vi "一体站流程自动启动.vi"(11 "参数":T1) -> ()   [LabVIEW 2016, in "PLC.lvlib"]
uses:
  PLC.lvlib
panel:
  out "s? t:f":enum16{"初始化", "采配水启动", "仪器操作", "反冲洗", "结束"}(ring)
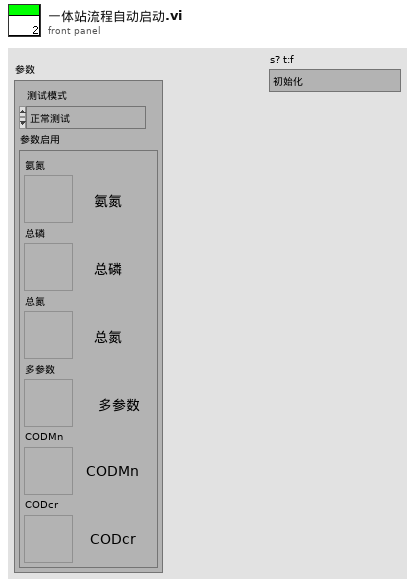
[diagram p1: front panel]
types:
  T1 = cluster{"测试模式":enum16{"正常测试", "集成干预"}, "参数启用":cluster{"氨氮":bool, "总磷":bool, "总氮":bool, "多参数":bool, "CODMn":bool, "CODcr":bool}}
  T2 = cluster{"命令":string, cluster{"starting address":u16, "holding register value":u16}}
  T3 = enum16{"启动测量", "标样核查", "零点核查", "跨度核查", "空白测试", "平行样测试", "加标回收", "空白校准", "标样校准", "初始化（清洗）", "停止测试", "仪器重启", "校时", "模式设置", "测量间隔设置"}
  T4 = cluster{"时间标识":timestamp, "设备":string, "日志信息":string, "流程参数":string}
  T5 = cluster{"测量模式":enum16{"水样测量", "标样核查", "零点核查", "跨度核查", "空白测试", "加标回收", "平行样", "校零", "校标"}}
  T6 = cluster{"时间标识":timestamp, "设备":string, "日志信息":string}
  T7 = enum16{"空闲", "水样测试", "标样核查", "零点核查", "跨度核查", "空白测试", "平行样测试", "加标回收", "空白校准", "标样校准", "初始化（清洗）"}
  T8 = cluster{"R0":i16, "R1":i16, "R2":i16, "R3":i16, "R4":i16, "R5":i16, "R6":i16, "R7":i16, "R8":i16, "R9":i16, "R10":i16, "R11":i16, "R12":i16, "R13":i16, "R14":i16, "R15":i16, "R16":i16, "R17":i16, "R18":i16, "R19":i16, "R20":i16, "R21":i16, "R22":i16, "R23":i16, "R24":i16, "R25":i16, "R26":i16, "R27":i16, "R28":i16, "R29":i16, "R30":i16, "R31":i16}
  T9 = cluster{"R100":i16, "R101":i16, "R102":i16, "R103":i16, "R104":i16, "R105":i16, "R106":i16, "R107":i16, "R108":i16, "R109":i16, "R110":i16, "R111":i16, "R112":i16, "R113":i16, "R114":i16, "R115":i16, "R116":i16, "R117":i16, "R118":i16, "R119":i16}
  T10 = enum32{"Bad", "Idle", "Run top level", "Running"}
  T11 = cluster{"氨氮":bool, "总磷":bool, "总氮":bool, "多参数":bool, "CODMn":bool, "CODcr":bool}
  T12 = cluster{"时间标识":timestamp, "参数":string, "集成干预测试浓度值":dbl, "集成干预前测试时间":timestamp, "集成干预前测试浓度值":dbl}
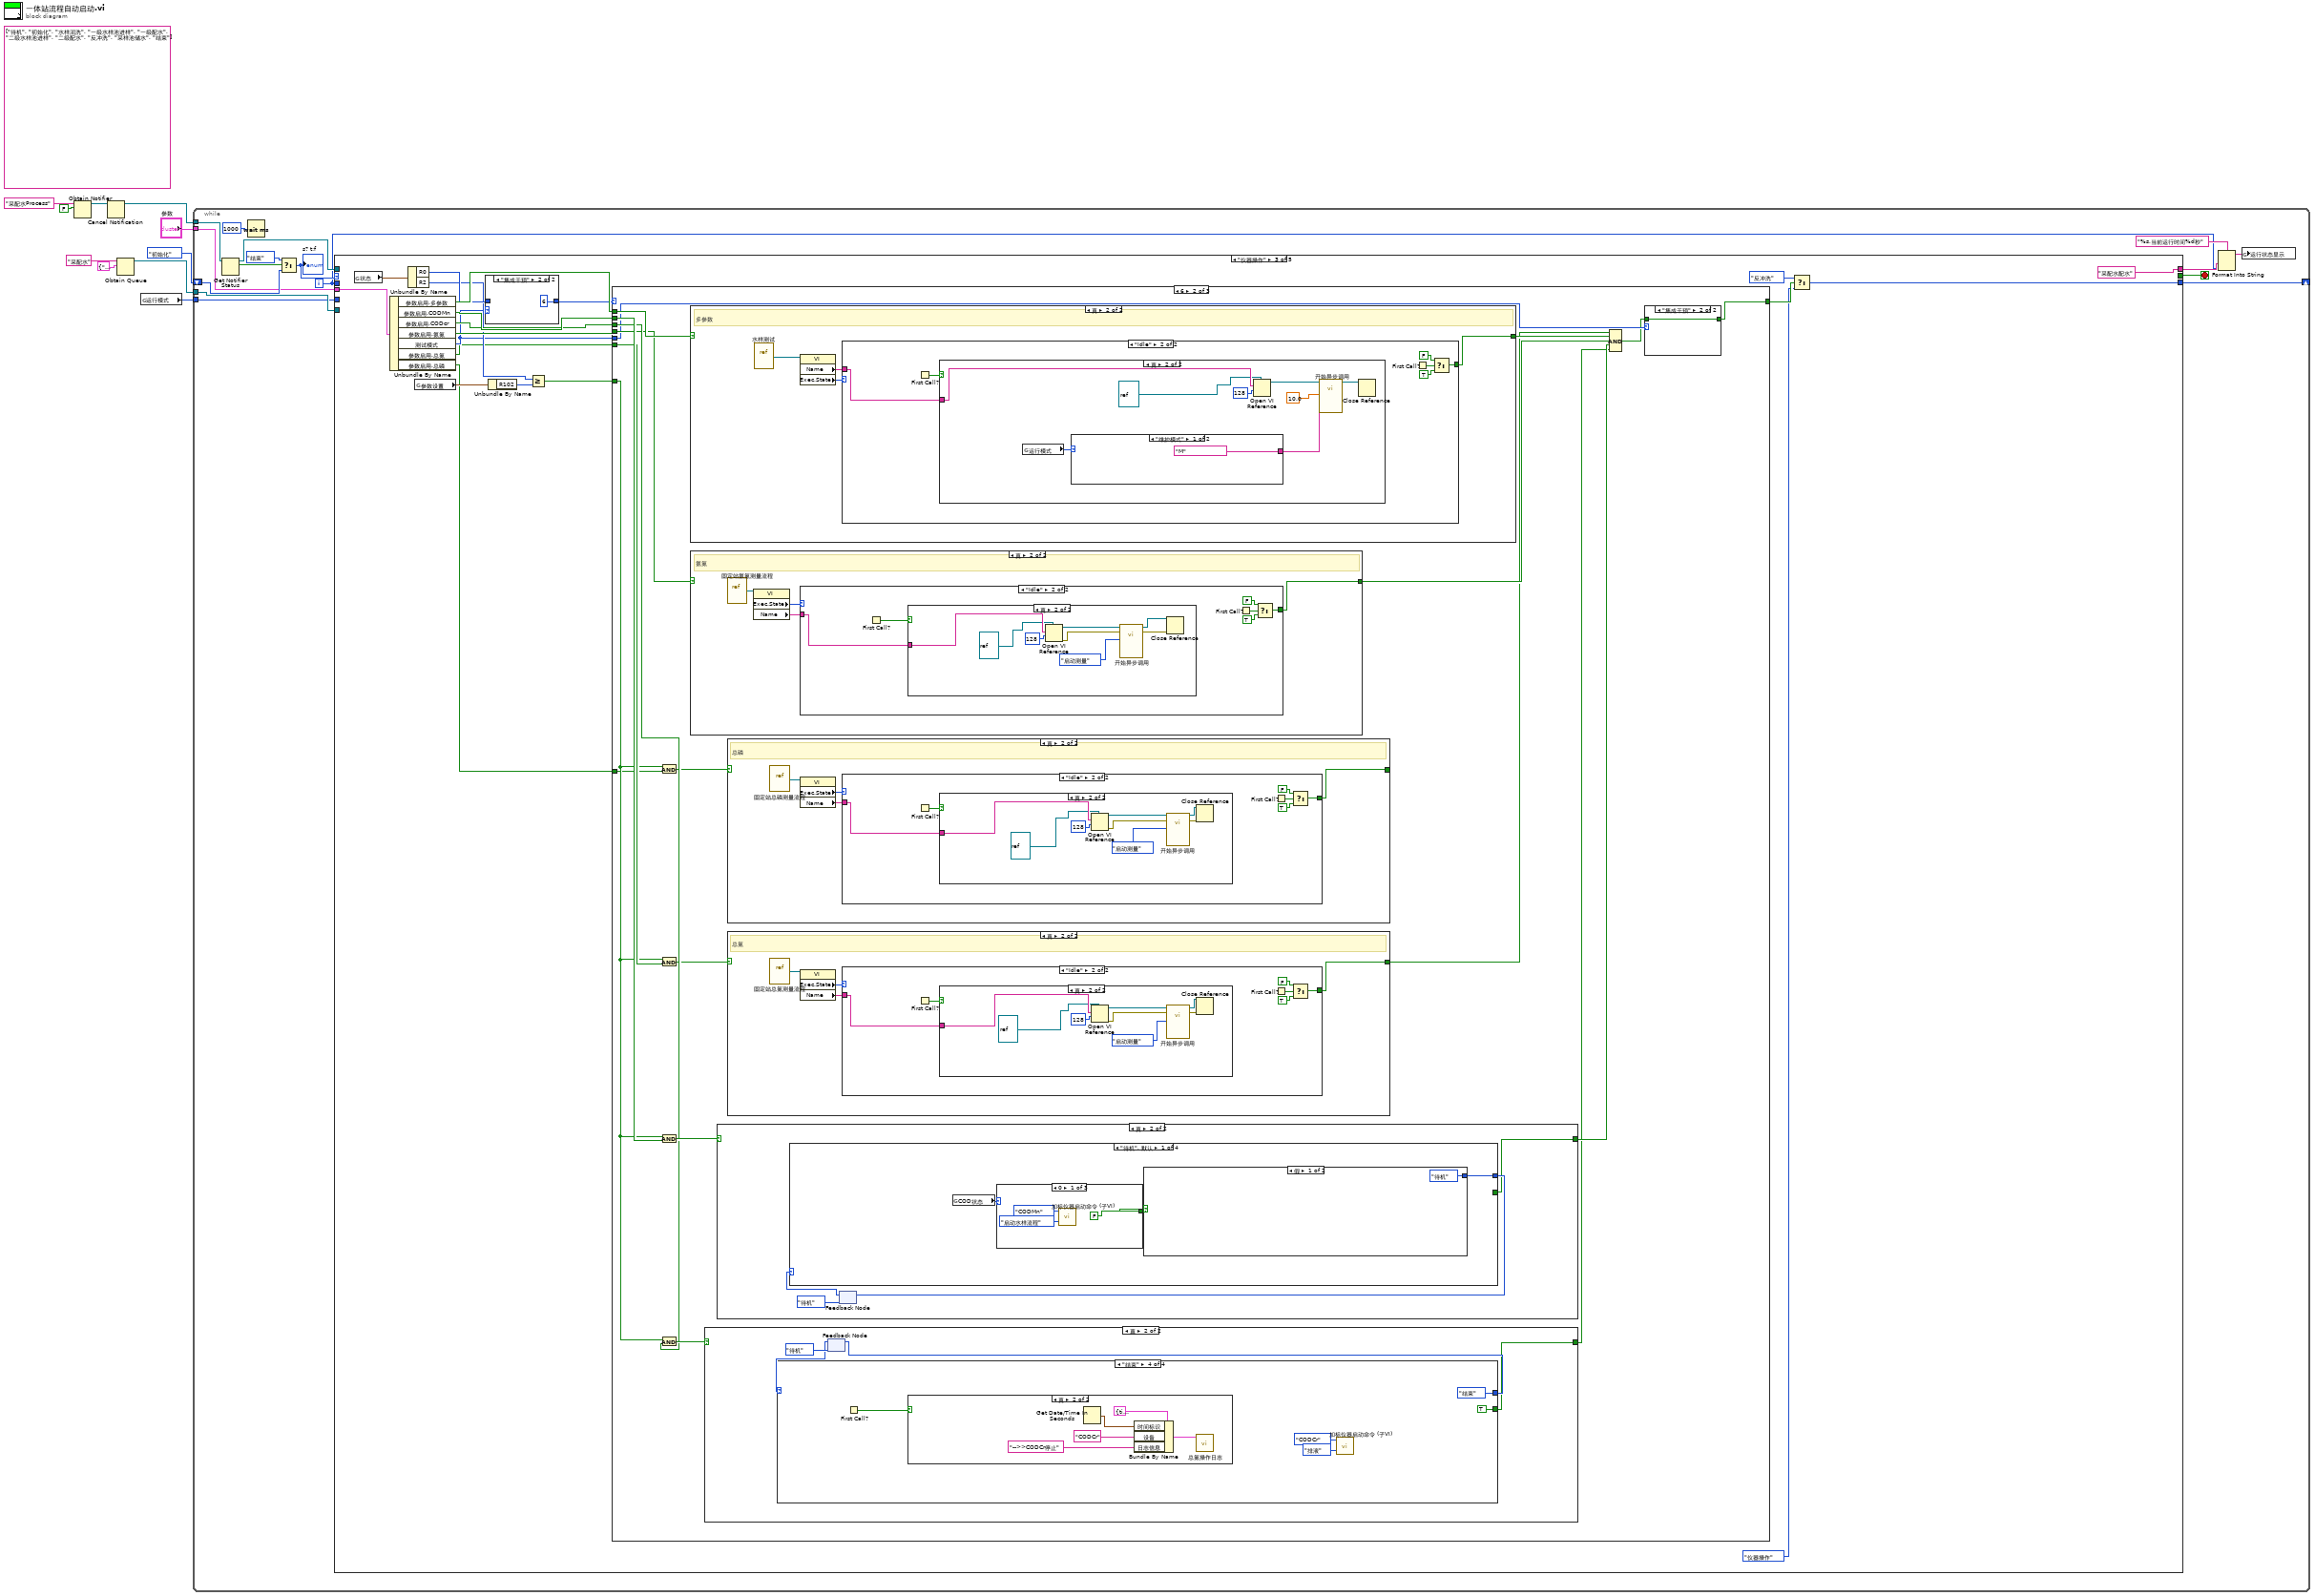
[diagram p0: block diagram]
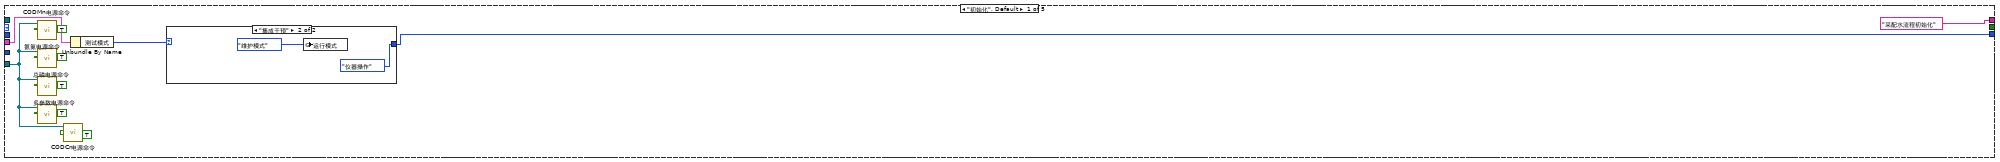
[diagram p2: hidden frame]
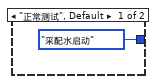
[diagram p3: hidden frame]
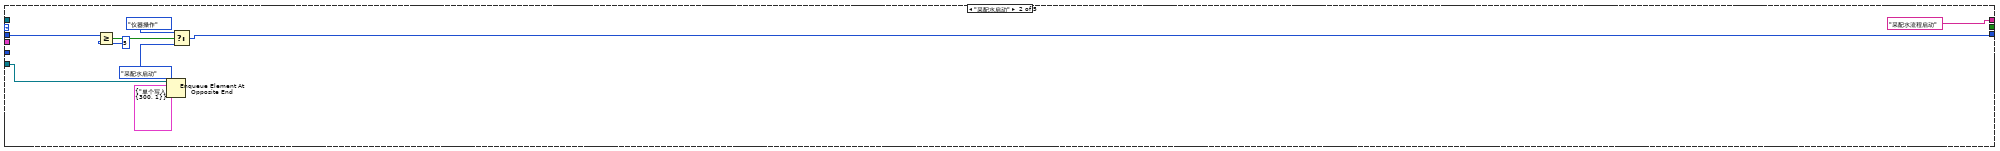
[diagram p4: hidden frame]
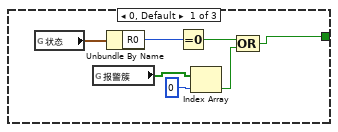
[diagram p6: hidden frame]
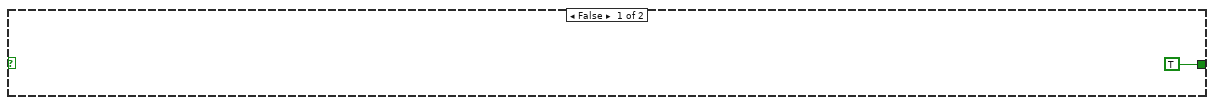
[diagram p7: hidden frame]
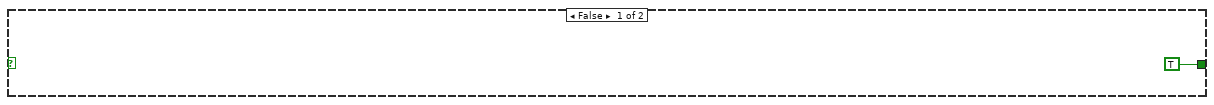
[diagram p10: hidden frame]
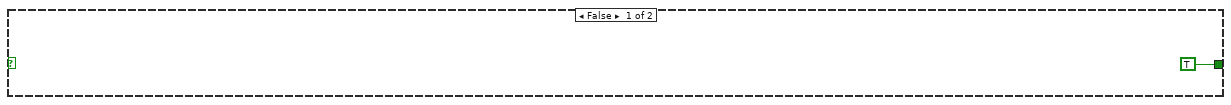
[diagram p14: hidden frame]
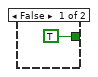
[diagram p17: hidden frame]
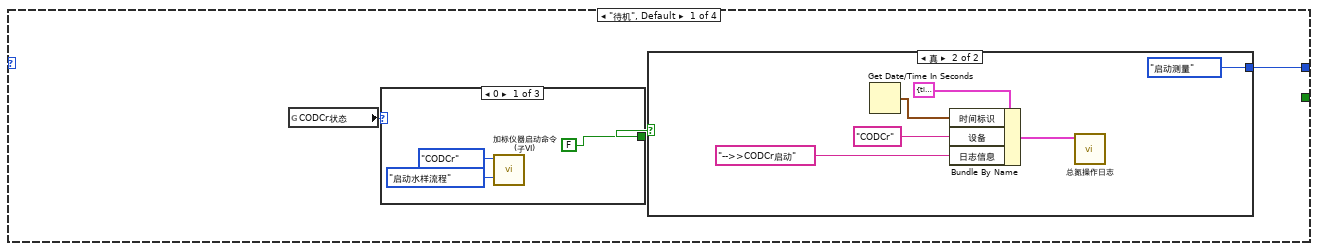
[diagram p18: hidden frame]
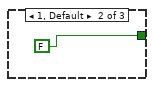
[diagram p19: hidden frame]
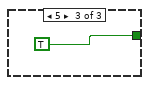
[diagram p20: hidden frame]
diagram:
  (unwired) string[][] [["待机"], ["初始化"], ["水样润洗"], ["一级水样池进样"], ["一级配水"], ["二级水样池进样"], ["二级配水"], ["反冲洗"], ["采样池储水"], ["结束"]] ("项名")
  n1 = Obtain Notifier(name (unnamed)="采配水Process" ("名称（未命名）"), notification data type=FALSE) -> (notifier out=w4:refnum<notifier>)  [unwired: 2 in, 2 out]
  n2 = Cancel Notification(0:w4) -> (8:w3:refnum<notifier>)  [unwired: 1 in, 2 out]
  n3 = Obtain Queue(name (unnamed)="采配水" ("名称（未命名）"), element data type=cluster{"命令":string, "数据":variant} {"命令"="", "数据"=variant}) -> (queue out=w7:refnum<queue>)  [unwired: 3 in, 2 out]
  n4 = global read "系统设置全局变量.vi" "运行模式"() -> (w1:enum16{"维护模式", "常规模式", "应急模式", "质控模式"})
  n5 = while {
    shift-right: [w23] -> _
    shift-left: enum16{"初始化", "采配水启动", "仪器操作", "反冲洗", "结束"}."初始化" ("枚举") -> [w19]
    tunnel: w7 -> [w26]
    tunnel: w3 -> [w22]
    tunnel: "参数" -> [w13]
    tunnel: w1 -> [w12]
    i -> [w11]
    stop <- w25 stop-if-true
    n6 = Get Notifier Status(notifier=w22) -> (notifier out=w14:refnum<notifier>, current notification=w21:bool)  [unwired: 1 in, 3 out]
    n7 = Wait (ms)(milliseconds to wait=u32 1000 ("等待时间（毫秒）")) -> ()  [unwired: 1 out]
    n8 = Select(t=enum16{"初始化", "采配水启动", "仪器操作", "反冲洗", "结束"}."结束" ("枚举"), s=w21, f=w19) -> (s? t:f=w18:enum16{"初始化", "采配水启动", "仪器操作", "反冲洗", "结束"})
    "s? t:f" <- w18
    n9 = case shown="\"仪器操作\"" w18 {
      tunnel: w26 -> [w31 w48 _ _ w473]
      tunnel: [_ _ _ _ TRUE] -> w25
      tunnel: [w30 w40 w63 w305 enum16{"初始化", "采配水启动", "仪器操作", "反冲洗", "结束"}."结束" ("枚举")] -> w23
      tunnel: ["采配水流程初始化" "采配水流程启动" "采配水配水" "等待测试完成" "采配水结束"] -> w15
      tunnel: w14 -> [_ _ _ _ w474]
      tunnel: w13 -> [w28 _ w66 w304 w470]
      tunnel: w12 -> [_ _ _ _ w469]
      tunnel: w11 -> [_ w46 _ _ _]
      frame "初始化", Default {
        n10 = call "CODMn电源命令.vi"("通电/断电"=TRUE, "队列"=w31) -> ()  [unwired: 9 in, 1 out]
        n11 = call "氨氮电源命令.vi"("通电/断电"=TRUE, "队列"=w31) -> ()  [unwired: 9 in, 1 out]
        n12 = call "总磷电源命令.vi"("通电/断电"=TRUE, "队列"=w31) -> ()  [unwired: 9 in, 1 out]
        n13 = call "多参数电源命令.vi"("通电/断电"=TRUE, "队列"=w31) -> ()  [unwired: 9 in, 1 out]
        n14 = call "CODCr电源命令.vi"("通电/断电"=TRUE, "队列"=w31) -> ()  [unwired: 9 in, 1 out]
        n15 = Unbundle By Name(w28) -> ("测试模式"=w27:enum16{"正常测试", "集成干预"})
        n16 = case shown="\"集成干预\"" w27 {
          tunnel: [enum16{"初始化", "采配水启动", "仪器操作", "反冲洗", "结束"}."采配水启动" ("枚举") enum16{"初始化", "采配水启动", "仪器操作", "反冲洗", "结束"}."仪器操作" ("枚举")] -> w30
          frame "正常测试", Default {
          }
          frame "集成干预" {
            n17 = global write "系统设置全局变量.vi" "运行模式"(enum16{"维护模式", "常规模式", "应急模式", "质控模式"}."维护模式" ("运行模式")) -> ()
          }
        }
      }
      frame "采配水启动" {
        n18 = Greater Or Equal?(x=w46, y=5) -> (x >= y?=w43:bool)
        n19 = Enqueue Element At Opposite End(queue=w48, element=T2 {"命令"="单个写入", {"starting address"=300, "holding register value"=1}} ("元素")) -> ()  [unwired: 2 in, 3 out]
        n20 = Select(t=enum16{"初始化", "采配水启动", "仪器操作", "反冲洗", "结束"}."仪器操作" ("枚举"), s=w43, f=enum16{"初始化", "采配水启动", "仪器操作", "反冲洗", "结束"}."采配水启动" ("枚举")) -> (s? t:f=w40:enum16{"初始化", "采配水启动", "仪器操作", "反冲洗", "结束"})
      }
      frame "仪器操作" {
        n21 = global read "采配水全局变量.vi" "状态"() -> (w68:T8)
        n22 = Unbundle By Name(w66) -> ("参数启用.多参数"=w61:bool, "参数启用.CODMn"=w60:bool, "参数启用.CODcr"=w59:bool, "参数启用.氨氮"=w58:bool, "测试模式"=w51:enum16{"正常测试", "集成干预"}, "参数启用.总氮"=w50:bool, "参数启用.总磷"=w49:bool)
        n23 = Unbundle By Name(w68) -> ("R0"=w57:i16, "R2"=w52:i16)
        n24 = global read "采配水全局变量.vi" "参数设置"() -> (w54:T9)
        n25 = case shown="\"集成干预\"" w51 {
          tunnel: w57 -> [w69 _]
          tunnel: [w69 i16 6 ("R0")] -> w56
          frame "正常测试", Default {
          }
          frame "集成干预" {
          }
        }
        n26 = Unbundle By Name(w54) -> ("R102"=w55:i16)
        n27 = Greater Or Equal?(x=w52, y=w55) -> (x >= y?=w53:bool)
        n28 = case shown="6" w56 {
          tunnel: [w72 w84 TRUE] -> w65
          tunnel: w61 -> [_ w96 _]
          tunnel: w60 -> [_ w95 _]
          tunnel: w59 -> [_ w92 _]
          tunnel: w58 -> [_ w91 _]
          tunnel: w53 -> [_ w80 _]
          tunnel: w51 -> [_ w86 _]
          tunnel: w50 -> [_ w83 _]
          tunnel: w49 -> [_ w79 _]
          frame 0, Default {
            n29 = global read "采配水全局变量.vi" "状态"() -> (w75:T8)
            n30 = global read "采配水全局变量.vi" "报警簇"() -> (w76:bool[])
            n31 = Unbundle By Name(w75) -> ("R0"=w74:i16)
            n32 = Equal To 0?(x=w74) -> (x = 0?=w77:bool)
            n33 = Index Array(array=w76, index=0 ("索引")) -> (element=w71:bool)
            n34 = Compound Arithmetic op=OR ("复合运算")(w77, w71) -> (w72:bool)
          }
          frame 6 {
            n35 = And(x=w80, y=w79) -> (x .and. y?=w78:bool)
            n36 = And(x=w80, y=w83) -> (x .and. y?=w82:bool)
            n37 = And(x=w80, y=w95) -> (x .and. y?=w94:bool)
            n38 = And(x=w80, y=w92) -> (x .and. y?=w93:bool)
            n39 = case shown="真" w96 {
              tunnel: [TRUE ("t") w281] -> w90
              frame False {
              }
              frame True {
                # "多参数"
                n40 = vi-ref "水样测试.vi"() -> (w283:refnum<vi>)
                n41 = property class="VI"(reference=w283) -> ("Name"=w282:string, "Exec.State"=w284:T10)  [unwired: 1 in, 2 out]
                n42 = case shown="\"Idle\"" w284 {
                  tunnel: w282 -> [_ w290]
                  tunnel: [_ w285] -> w281
                  frame "Bad", Default {
                  }
                  frame "Idle" {
                    n43 = First Call?() -> (First Call?: T/F=w289:bool)
                    n44 = case shown="真" w289 {
                      tunnel: w290 -> [_ w297]
                      frame False {
                      }
                      frame True {
                        n45 = global read "系统设置全局变量.vi" "运行模式"() -> (w294:enum16{"维护模式", "常规模式", "应急模式", "质控模式"})
                        n46 = case shown="\"维护模式\"" w294 {
                          tunnel: ["M" ("数据标记表") "N" ("数据标记表")] -> w293
                          frame "维护模式" {
                          }
                          frame "常规模式", Default {
                          }
                        }
                        n47 = Open VI Reference(type specifier VI Refnum (for type only)=refnum<vi> refnum, vi path=w297, options=128 ("选项")) -> (vi reference=w296:refnum<vi>)  [unwired: 3 in, 1 out]
                        n48 = call-by-ref "开始异步调用"(reference=w296, "数据标记表"=w293, "水样测试时间"=10.0) -> (reference out=w295:refnum<vi>)  [unwired: 11 in, 1 out]
                        n49 = Close Reference(reference=w295) -> ()  [unwired: 1 in, 1 out]
                      }
                    }
                    n50 = First Call?() -> (First Call?: T/F=w288:bool)
                    n51 = Select(t=FALSE, s=w288, f=TRUE) -> (s? t:f=w285:bool)
                  }
                }
              }
            }
            n52 = case "条件结构" shown="真" w91 {
              tunnel: [TRUE ("t") w137] -> w89
              frame False {
              }
              frame True {
                # "氨氮"
                n53 = vi-ref "固定站氨氮测量流程.vi"() -> (w140:refnum<vi>)
                n54 = property class="VI"(reference=w140) -> ("Exec.State"=w139:T10, "Name"=w138:string)  [unwired: 1 in, 2 out]
                n55 = case shown="\"Idle\"" w139 {
                  tunnel: w138 -> [_ w146]
                  tunnel: [_ w141] -> w137
                  frame "Bad", Default {
                  }
                  frame "Idle" {
                    n56 = First Call?() -> (First Call?: T/F=w145:bool)
                    n57 = case shown="真" w145 {
                      tunnel: w146 -> [_ w151]
                      frame False {
                      }
                      frame True {
                        n58 = Open VI Reference(type specifier VI Refnum (for type only)=refnum<vi> refnum, vi path=w151, options=128 ("选项")) -> (vi reference=w149:refnum<vi>, error out=w152:errorcluster)  [unwired: 3 in]
                        n59 = call-by-ref "开始异步调用"(reference=w149, error in=w152, "控制命令"=T3."启动测量") -> (reference out=w153:refnum<vi>, error out=w154:errorcluster)  [unwired: 11 in]
                        n60 = Close Reference(reference=w153, error in (no error)=w154) -> ()  [unwired: 1 out]
                      }
                    }
                    n61 = First Call?() -> (First Call?: T/F=w144:bool)
                    n62 = Select(t=FALSE, s=w144, f=TRUE) -> (s? t:f=w141:bool)
                  }
                }
              }
            }
            n63 = case shown="真" w93 {
              tunnel: [TRUE w156] -> w87
              frame False {
              }
              frame True {
                n64 = feedback #1(enum16{"待机", "启动测量", "测量中", "结束"}."待机") -> (w158:enum16{"待机", "启动测量", "测量中", "结束"})
                n65 = case shown="\"结束\"" w158 {
                  tunnel: [w162 w183 w203 enum16{"待机", "启动测量", "测量中", "结束"}."结束"] -> w157
                  tunnel: [_ _ _ TRUE] -> w156
                  frame "待机", Default {
                    n66 = global read "加标回收状态全局变量.vi" "CODCr状态"() -> (w161:u16)
                    n67 = case shown="0" w161 {
                      tunnel: [FALSE ("s") FALSE ("s") TRUE ("s")] -> w160
                      frame 0 {
                        n68 = call "加标仪器启动命令 (子VI).vi"("启动命令"=enum16{"启动水样流程", "启动加标流程", "排液", "停止", "柱塞泵启动"}."启动水样流程", "仪器"=enum16{"", "氨氮", "总磷", "总氮", "CODMn", "CODCr"}."CODCr") -> ()  [unwired: 9 in, 1 out]
                      }
                      frame 1, Default {
                      }
                      frame 5 {
                      }
                    }
                    n69 = case shown="真" w160 {
                      tunnel: [enum16{"待机", "启动测量", "测量中", "结束"}."待机" enum16{"待机", "启动测量", "测量中", "结束"}."启动测量"] -> w162
                      frame False {
                      }
                      frame True {
                        n70 = Get Date/Time In Seconds() -> (seconds since 1Jan1904=w173:timestamp)
                        n71 = Bundle By Name(cluster=T4 {"时间标识"=timestamp(0 s since 1904-01-01), "设备"="", "日志信息"="", "流程参数"=""} ("data in"), "时间标识"=w173, "设备"="CODCr", "日志信息"="-->>CODCr启动") -> (w169:T4)
                        n72 = call "总氮操作日志.vi"("data in"=w169) -> ()  [unwired: 11 in]
                      }
                    }
                  }
                  frame "启动测量" {
                    # "CODcr"
                    n73 = feedback #2() -> (w179:i32)  [unwired: 1 in]
                    n74 = Increment(x=w179) -> (x+1=w180:i32)
                    n75 = First Call?() -> (First Call?: T/F=w178:bool)
                    n76 = call "CODCr启动命令 (子VI).vi"("启动测量模式"=T5 {"测量模式"=enum."水样测量"}) -> ()  [unwired: 11 in]
                    n77 = Select(t=0, s=w178, f=w180) -> (s? t:f=w181:i32)
                    n78 = feedback-in #2(w181) -> ()
                    n79 = Greater Or Equal?(x=w181, y=60) -> (x >= y?=w176:bool)
                    n80 = case shown="真" w176 {
                      tunnel: [w184 enum16{"待机", "启动测量", "测量中", "结束"}."结束"] -> w183
                      frame False {
                        n81 = global read "CODcr全局变量.vi" "工作状态"() -> (w185:T7)
                        n82 = Not Equal To 0?(x=w185) -> (x != 0?=w186:bool)
                        n83 = Select(t=enum16{"待机", "启动测量", "测量中", "结束"}."测量中", s=w186, f=enum16{"待机", "启动测量", "测量中", "结束"}."启动测量") -> (s? t:f=w184:enum16{"待机", "启动测量", "测量中", "结束"})
                      }
                      frame True {
                        n84 = Get Date/Time In Seconds() -> (seconds since 1Jan1904=w195:timestamp)
                        n85 = Bundle By Name(cluster=T6 {"时间标识"=timestamp(0 s since 1904-01-01), "设备"="", "日志信息"=""} ("data in"), "时间标识"=w195, "设备"="CODCr", "日志信息"="CODCr启动失败") -> (w189:T6)
                        n86 = call "报警信息字段定义.vi"("table输入"="报警信息", "data in"=w189) -> ("table输出"=w192:string, "columns"=w193:string[], "data out"=w194:T6)  [unwired: 7 in]
                        n87 = call "插入数据.vi"("data"=w194, "columns"=w193, "database"="database3.mdb", "table"=w192) -> ()  [unwired: 7 in, 1 out]
                      }
                    }
                  }
                  frame "测量中" {
                    n88 = global read "CODcr全局变量.vi" "工作状态"() -> (w202:T7)
                    n89 = Equal?(x=w202, y=T7."空闲" ("工作状态")) -> (x = y?=w201:bool)
                    n90 = case shown="假" w201 {
                      tunnel: [w204 enum16{"待机", "启动测量", "测量中", "结束"}."结束"] -> w203
                      frame False {
                        n91 = flat-sequence {
                          tunnel: [enum16{"待机", "启动测量", "测量中", "结束"}."测量中"] -> w204
                          frame #0 {
                            n92 = Wait (ms)(milliseconds to wait=u32 1000 ("等待时间（毫秒）")) -> ()  [unwired: 1 out]
                          }
                          frame #1 {
                          }
                        }
                      }
                      frame True {
                      }
                    }
                  }
                  frame "结束" {
                    n93 = First Call?() -> (First Call?: T/F=w210:bool)
                    n94 = case shown="真" w210 {
                      frame False {
                      }
                      frame True {
                        n95 = Get Date/Time In Seconds() -> (seconds since 1Jan1904=w217:timestamp)
                        n96 = Bundle By Name(cluster=T4 {"时间标识"=timestamp(0 s since 1904-01-01), "设备"="", "日志信息"="", "流程参数"=""} ("data in"), "时间标识"=w217, "设备"="CODCr", "日志信息"="-->>CODCr停止") -> (w213:T4)
                        n97 = call "总氮操作日志.vi"("data in"=w213) -> ()  [unwired: 11 in]
                      }
                    }
                    n98 = call "加标仪器启动命令 (子VI).vi"("启动命令"=enum16{"启动水样流程", "启动加标流程", "排液", "停止", "柱塞泵启动"}."排液", "仪器"=enum16{"", "氨氮", "总磷", "总氮", "CODMn", "CODCr"}."CODCr") -> ()  [unwired: 9 in, 1 out]
                  }
                }
                n99 = feedback-in #1(w157) -> ()
              }
            }
            n100 = case shown="真" w94 {
              tunnel: [TRUE w219] -> w88
              frame False {
              }
              frame True {
                n101 = feedback #3(enum16{"待机", "启动测量", "测量中", "结束"}."待机") -> (w221:enum16{"待机", "启动测量", "测量中", "结束"})
                n102 = case shown="\"待机\", 默认" w221 {
                  tunnel: [w225 w246 w265 enum16{"待机", "启动测量", "测量中", "结束"}."结束"] -> w220
                  tunnel: [_ _ _ TRUE] -> w219
                  frame "待机", Default {
                    n103 = global read "加标回收状态全局变量.vi" "COD状态"() -> (w224:u16)
                    n104 = case shown="0" w224 {
                      tunnel: [FALSE ("s") FALSE ("s") TRUE ("s")] -> w223
                      frame 0 {
                        n105 = call "加标仪器启动命令 (子VI).vi"("启动命令"=enum16{"启动水样流程", "启动加标流程", "排液", "停止", "柱塞泵启动"}."启动水样流程", "仪器"=enum16{"", "氨氮", "总磷", "总氮", "CODMn", "CODCr"}."CODMn") -> ()  [unwired: 9 in, 1 out]
                      }
                      frame 1, Default {
                      }
                      frame 5 {
                      }
                    }
                    n106 = case shown="假" w223 {
                      tunnel: [enum16{"待机", "启动测量", "测量中", "结束"}."待机" enum16{"待机", "启动测量", "测量中", "结束"}."启动测量"] -> w225
                      frame False {
                      }
                      frame True {
                        n107 = Get Date/Time In Seconds() -> (seconds since 1Jan1904=w236:timestamp)
                        n108 = Bundle By Name(cluster=T4 {"时间标识"=timestamp(0 s since 1904-01-01), "设备"="", "日志信息"="", "流程参数"=""} ("data in"), "时间标识"=w236, "设备"="CODMn", "日志信息"="-->>CODMn启动") -> (w232:T4)
                        n109 = call "总氮操作日志.vi"("data in"=w232) -> ()  [unwired: 11 in]
                      }
                    }
                  }
                  frame "启动测量" {
                    # "CODMn"
                    n110 = feedback #4() -> (w242:i32)  [unwired: 1 in]
                    n111 = Increment(x=w242) -> (x+1=w243:i32)
                    n112 = First Call?() -> (First Call?: T/F=w241:bool)
                    n113 = call "CODMn启动命令 (子VI).vi"("启动测量模式"=T5 {"测量模式"=enum."水样测量"}) -> ()  [unwired: 11 in]
                    n114 = Select(t=0, s=w241, f=w243) -> (s? t:f=w244:i32)
                    n115 = feedback-in #4(w244) -> ()
                    n116 = Greater Or Equal?(x=w244, y=60) -> (x >= y?=w239:bool)
                    n117 = case shown="假" w239 {
                      tunnel: [w248 enum16{"待机", "启动测量", "测量中", "结束"}."结束"] -> w246
                      frame False {
                        n118 = global read "运行时序全局变量.vi" "多列列表框"() -> (w247:i32)
                        n119 = Not Equal To 0?(x=w247) -> (x != 0?=w249:bool)
                        n120 = Select(t=enum16{"待机", "启动测量", "测量中", "结束"}."测量中", s=w249, f=enum16{"待机", "启动测量", "测量中", "结束"}."启动测量") -> (s? t:f=w248:enum16{"待机", "启动测量", "测量中", "结束"})
                      }
                      frame True {
                        n121 = Get Date/Time In Seconds() -> (seconds since 1Jan1904=w258:timestamp)
                        n122 = Bundle By Name(cluster=T6 {"时间标识"=timestamp(0 s since 1904-01-01), "设备"="", "日志信息"=""} ("data in"), "时间标识"=w258, "设备"="CODMn", "日志信息"="CODMn启动失败") -> (w252:T6)
                        n123 = call "报警信息字段定义.vi"("table输入"="报警信息", "data in"=w252) -> ("table输出"=w255:string, "columns"=w256:string[], "data out"=w257:T6)  [unwired: 7 in]
                        n124 = call "插入数据.vi"("data"=w257, "columns"=w256, "database"="database3.mdb", "table"=w255) -> ()  [unwired: 7 in, 1 out]
                      }
                    }
                  }
                  frame "测量中" {
                    n125 = global read "运行时序全局变量.vi" "多列列表框"() -> (w264:i32)
                    n126 = Equal To 0?(x=w264) -> (x = 0?=w263:bool)
                    n127 = case shown="假" w263 {
                      tunnel: [w266 enum16{"待机", "启动测量", "测量中", "结束"}."结束"] -> w265
                      frame False {
                        n128 = flat-sequence {
                          tunnel: [enum16{"待机", "启动测量", "测量中", "结束"}."测量中"] -> w266
                          frame #0 {
                            n129 = Wait (ms)(milliseconds to wait=u32 1000 ("等待时间（毫秒）")) -> ()  [unwired: 1 out]
                          }
                          frame #1 {
                          }
                        }
                      }
                      frame True {
                      }
                    }
                  }
                  frame "结束" {
                    n130 = call "加标仪器启动命令 (子VI).vi"("启动命令"=enum16{"启动水样流程", "启动加标流程", "排液", "停止", "柱塞泵启动"}."排液", "仪器"=enum16{"", "氨氮", "总磷", "总氮", "CODMn", "CODCr"}."CODMn") -> ()  [unwired: 9 in, 1 out]
                    n131 = First Call?() -> (First Call?: T/F=w272:bool)
                    n132 = case shown="真" w272 {
                      frame False {
                      }
                      frame True {
                        n133 = Get Date/Time In Seconds() -> (seconds since 1Jan1904=w279:timestamp)
                        n134 = Bundle By Name(cluster=T4 {"时间标识"=timestamp(0 s since 1904-01-01), "设备"="", "日志信息"="", "流程参数"=""} ("data in"), "时间标识"=w279, "设备"="CODMn", "日志信息"="-->>CODMn停止") -> (w275:T4)
                        n135 = call "总氮操作日志.vi"("data in"=w275) -> ()  [unwired: 11 in]
                      }
                    }
                  }
                }
                n136 = feedback-in #3(w220) -> ()
              }
            }
            n137 = case "条件结构" shown="真" w78 {
              tunnel: [TRUE ("t") w98] -> _
              frame False {
              }
              frame True {
                # "总磷"
                n138 = vi-ref "固定站总磷测量流程.vi"() -> (w101:refnum<vi>)
                n139 = property class="VI"(reference=w101) -> ("Exec.State"=w100:T10, "Name"=w99:string)  [unwired: 1 in, 2 out]
                n140 = case shown="\"Idle\"" w100 {
                  tunnel: w99 -> [_ w107]
                  tunnel: [_ w102] -> w98
                  frame "Bad", Default {
                  }
                  frame "Idle" {
                    n141 = First Call?() -> (First Call?: T/F=w106:bool)
                    n142 = case shown="真" w106 {
                      tunnel: w107 -> [_ w112]
                      frame False {
                      }
                      frame True {
                        n143 = Open VI Reference(type specifier VI Refnum (for type only)=refnum<vi> refnum, vi path=w112, options=128 ("选项")) -> (vi reference=w110:refnum<vi>, error out=w113:errorcluster)  [unwired: 3 in]
                        n144 = call-by-ref "开始异步调用"(reference=w110, error in=w113, "控制命令"=T3."启动测量") -> (reference out=w114:refnum<vi>, error out=w115:errorcluster)  [unwired: 11 in]
                        n145 = Close Reference(reference=w114, error in (no error)=w115) -> ()  [unwired: 1 out]
                      }
                    }
                    n146 = First Call?() -> (First Call?: T/F=w105:bool)
                    n147 = Select(t=FALSE, s=w105, f=TRUE) -> (s? t:f=w102:bool)
                  }
                }
              }
            }
            n148 = case "条件结构" shown="真" w82 {
              tunnel: [TRUE ("t") w117] -> w81
              frame False {
              }
              frame True {
                # "总氮"
                n149 = vi-ref "固定站总氮测量流程.vi"() -> (w120:refnum<vi>)
                n150 = property class="VI"(reference=w120) -> ("Exec.State"=w119:T10, "Name"=w118:string)  [unwired: 1 in, 2 out]
                n151 = case shown="\"Idle\"" w119 {
                  tunnel: w118 -> [_ w126]
                  tunnel: [_ w121] -> w117
                  frame "Bad", Default {
                  }
                  frame "Idle" {
                    n152 = First Call?() -> (First Call?: T/F=w125:bool)
                    n153 = case shown="真" w125 {
                      tunnel: w126 -> [_ w131]
                      frame False {
                      }
                      frame True {
                        n154 = Open VI Reference(type specifier VI Refnum (for type only)=refnum<vi> refnum, vi path=w131, options=128 ("选项")) -> (vi reference=w129:refnum<vi>, error out=w132:errorcluster)  [unwired: 3 in]
                        n155 = call-by-ref "开始异步调用"(reference=w129, error in=w132, "控制命令"=T3."启动测量") -> (reference out=w133:refnum<vi>, error out=w134:errorcluster)  [unwired: 11 in]
                        n156 = Close Reference(reference=w133, error in (no error)=w134) -> ()  [unwired: 1 out]
                      }
                    }
                    n157 = First Call?() -> (First Call?: T/F=w124:bool)
                    n158 = Select(t=FALSE, s=w124, f=TRUE) -> (s? t:f=w121:bool)
                  }
                }
              }
            }
            n159 = Compound Arithmetic op=AND ("复合运算")(w81, w90, w89, w88, w87) -> (w85:bool)
            n160 = case shown="\"集成干预\"" w86 {
              tunnel: w85 -> [_ w135]
              tunnel: [_ w135] -> w84
              frame "正常测试", Default {
              }
              frame "集成干预" {
              }
            }
          }
          frame 7..9 {
          }
        }
        n161 = Select(t=enum16{"初始化", "采配水启动", "仪器操作", "反冲洗", "结束"}."反冲洗" ("枚举"), s=w65, f=enum16{"初始化", "采配水启动", "仪器操作", "反冲洗", "结束"}."仪器操作" ("枚举")) -> (s? t:f=w63:enum16{"初始化", "采配水启动", "仪器操作", "反冲洗", "结束"})
      }
      frame "反冲洗" {
        n162 = First Call?() -> (First Call?: T/F=w302:bool)
        n163 = case shown="真" w302 {
          tunnel: w304 -> [_ w313]
          frame False {
          }
          frame True {
            n164 = Unbundle By Name(w313) -> ("测试模式"=w312:enum16{"正常测试", "集成干预"}, "参数启用"=w311:T11)
            n165 = case shown="\"正常测试\", 默认" w312 {
              tunnel: w311 -> [w316 w402]
              frame "正常测试", Default {
                n166 = global read "系统设置全局变量.vi" "运行模式"() -> (w314:enum16{"维护模式", "常规模式", "应急模式", "质控模式"})
                n167 = global read "采配水全局变量.vi" "报警簇"() -> (w321:bool[])
                n168 = case shown="\"维护模式\"" w314 {
                  tunnel: ["M" ("table") "N" ("table")] -> w315
                  frame "维护模式" {
                  }
                  frame "常规模式", Default {
                  }
                }
                n169 = Index Array(array=w321, index #1=0 ("索引"), index #2=11 ("索引")) -> (element #1=w318:bool, element #2=w317:bool)
                n170 = case shown="真" w318 {
                  tunnel: w317 -> [w327 _]
                  tunnel: w316 -> [w326 w341]
                  tunnel: w315 -> [w324 w335]
                  frame False {
                    n171 = Unbundle By Name(w326) -> ("氨氮"=w325:bool)
                    n172 = case shown="真" w327 {
                      tunnel: w325 -> [_ w329]
                      tunnel: w324 -> [_ w328]
                      frame False {
                      }
                      frame True {
                        n173 = case shown="真" w329 {
                          tunnel: w328 -> [_ w330]
                          tunnel: [_ w331] -> _
                          frame False {
                          }
                          frame True {
                            n174 = call "取水点无水样数据存储.vi"("数据标识"="lw", "数据类型"=w330, "table"="氨氮") -> ("error out"=w331:errorcluster)  [unwired: 8 in]
                          }
                        }
                      }
                    }
                  }
                  frame True {
                    n175 = Unbundle By Name(w341) -> ("氨氮"=w340:bool, "CODMn"=w339:bool, "CODcr"=w338:bool, "多参数"=w337:bool, "总氮"=w336:bool, "总磷"=w334:bool)
                    n176 = case shown="真" w340 {
                      tunnel: w335 -> [_ w392]
                      tunnel: [_ w393] -> _
                      frame False {
                      }
                      frame True {
                        n177 = call "取水点无水样数据存储.vi"("数据标识"="Z", "数据类型"=w392, "table"="氨氮") -> ("error out"=w393:errorcluster)  [unwired: 8 in]
                      }
                    }
                    n178 = case shown="真" w336 {
                      tunnel: w335 -> [_ w345]
                      frame False {
                      }
                      frame True {
                        n179 = call "取水点无水样数据存储.vi"("数据标识"="Z", "数据类型"=w345, "table"="总氮") -> ()  [unwired: 8 in, 1 out]
                      }
                    }
                    n180 = case shown="真" w339 {
                      tunnel: w335 -> [_ w389]
                      tunnel: [_ w388] -> _
                      frame False {
                      }
                      frame True {
                        n181 = call "取水点无水样数据存储.vi"("数据标识"="Z", "数据类型"=w389, "table"="CODMn") -> ("error out"=w388:errorcluster)  [unwired: 8 in]
                      }
                    }
                    n182 = case shown="真" w338 {
                      tunnel: w335 -> [_ w385]
                      tunnel: [_ w384] -> _
                      frame False {
                      }
                      frame True {
                        n183 = call "取水点无水样数据存储.vi"("数据标识"="Z", "数据类型"=w385, "table"="CODCr") -> ("error out"=w384:errorcluster)  [unwired: 8 in]
                      }
                    }
                    n184 = case shown="真" w337 {
                      tunnel: w335 -> [_ w355]
                      frame False {
                      }
                      frame True {
                        n185 = global read "断电保存变量.vi" "Cond"() -> (w349:bool)
                        n186 = global read "断电保存变量.vi" "Turb"() -> (w350:bool)
                        n187 = global read "断电保存变量.vi" "DO"() -> (w351:bool)
                        n188 = global read "断电保存变量.vi" "pH"() -> (w352:bool)
                        n189 = global read "断电保存变量.vi" "Temp"() -> (w353:bool)
                        n190 = case shown="真" w352 {
                          tunnel: w355 -> [_ w377]
                          tunnel: [_ w376] -> _
                          frame False {
                          }
                          frame True {
                            n191 = call "取水点无水样数据存储.vi"("数据标识"="Z", "数据类型"=w377, "table"="pH") -> ("error out"=w376:errorcluster)  [unwired: 8 in]
                          }
                        }
                        n192 = case shown="真" w351 {
                          tunnel: w355 -> [_ w373]
                          tunnel: [_ w372] -> _
                          frame False {
                          }
                          frame True {
                            n193 = call "取水点无水样数据存储.vi"("数据标识"="Z", "数据类型"=w373, "table"="DO") -> ("error out"=w372:errorcluster)  [unwired: 8 in]
                          }
                        }
                        n194 = case shown="真" w350 {
                          tunnel: w355 -> [_ w365]
                          tunnel: [_ w364] -> _
                          frame False {
                          }
                          frame True {
                            n195 = call "取水点无水样数据存储.vi"("数据标识"="Z", "数据类型"=w365, "table"="浊度") -> ("error out"=w364:errorcluster)  [unwired: 8 in]
                          }
                        }
                        n196 = case shown="真" w349 {
                          tunnel: w355 -> [_ w369]
                          tunnel: [_ w368] -> _
                          frame False {
                          }
                          frame True {
                            n197 = call "取水点无水样数据存储.vi"("数据标识"="Z", "数据类型"=w369, "table"="比电导率") -> ("error out"=w368:errorcluster)  [unwired: 8 in]
                          }
                        }
                        n198 = case shown="真" FALSE {
                          tunnel: w355 -> [_ w357]
                          tunnel: [_ w356] -> _
                          frame False {
                          }
                          frame True {
                            n199 = call "取水点无水样数据存储.vi"("数据标识"="Z", "数据类型"=w357, "table"="藻密度") -> ("error out"=w356:errorcluster)  [unwired: 8 in]
                          }
                        }
                        n200 = global read "断电保存变量.vi" "叶绿素a启用"() -> (w348:bool)
                        n201 = case shown="真" w353 {
                          tunnel: w355 -> [_ w381]
                          tunnel: [_ w380] -> _
                          frame False {
                          }
                          frame True {
                            n202 = call "取水点无水样数据存储.vi"("数据标识"="Z", "数据类型"=w381, "table"="水温") -> ("error out"=w380:errorcluster)  [unwired: 8 in]
                          }
                        }
                        n203 = case shown="真" w348 {
                          tunnel: w355 -> [_ w361]
                          tunnel: [_ w360] -> _
                          frame False {
                          }
                          frame True {
                            n204 = call "取水点无水样数据存储.vi"("数据标识"="Z", "数据类型"=w361, "table"="叶绿素") -> ("error out"=w360:errorcluster)  [unwired: 8 in]
                          }
                        }
                      }
                    }
                    n205 = case shown="真" w334 {
                      tunnel: [_ w342] -> _
                      frame False {
                      }
                      frame True {
                        n206 = call "取水点无水样数据存储.vi"("数据标识"="Z", "table"="总磷") -> ("error out"=w342:errorcluster)  [unwired: 9 in]
                      }
                    }
                  }
                }
              }
              frame "集成干预" {
                n207 = Unbundle By Name(w402) -> ("总磷"=w396:bool, "总氮"=w397:bool, "氨氮"=w401:bool, "CODMn"=w400:bool, "CODcr"=w399:bool, "多参数"=w398:bool)
                n208 = case shown="真" w396 {
                  frame False {
                  }
                  frame True {
                    n209 = call "获取最近两组水样测试数据.vi"("table"="总磷") -> ("error out"=w408:errorcluster, "存储变量"=w407:T12)  [unwired: 9 in]
                    n210 = call "集成干预测试数据存储.vi"("error in (no error)"=w408, "存储变量"=w407) -> ()  [unwired: 9 in, 1 out]
                  }
                }
                n211 = case shown="真" w397 {
                  frame False {
                  }
                  frame True {
                    n212 = call "获取最近两组水样测试数据.vi"("table"="总氮") -> ("error out"=w405:errorcluster, "存储变量"=w404:T12)  [unwired: 9 in]
                    n213 = call "集成干预测试数据存储.vi"("error in (no error)"=w405, "存储变量"=w404) -> ()  [unwired: 9 in, 1 out]
                  }
                }
                n214 = case shown="真" w401 {
                  frame False {
                  }
                  frame True {
                    n215 = call "获取最近两组水样测试数据.vi"("table"="氨氮") -> ("error out"=w466:errorcluster, "存储变量"=w467:T12)  [unwired: 9 in]
                    n216 = call "集成干预测试数据存储.vi"("error in (no error)"=w466, "存储变量"=w467) -> ("error out"=w462:errorcluster)  [unwired: 9 in]
                    n217 = call "获取最近两组水样测试数据.vi"("error in (no error)"=w462, "table"="总磷") -> ("error out"=w465:errorcluster, "存储变量"=w464:T12)  [unwired: 8 in]
                    n218 = call "集成干预测试数据存储.vi"("error in (no error)"=w465, "存储变量"=w464) -> ()  [unwired: 9 in, 1 out]
                  }
                }
                n219 = case shown="真" w400 {
                  frame False {
                  }
                  frame True {
                    n220 = call "获取最近两组水样测试数据.vi"("table"="CODMn") -> ("error out"=w459:errorcluster, "存储变量"=w460:T12)  [unwired: 9 in]
                    n221 = call "集成干预测试数据存储.vi"("error in (no error)"=w459, "存储变量"=w460) -> ()  [unwired: 9 in, 1 out]
                  }
                }
                n222 = case shown="真" w399 {
                  frame False {
                  }
                  frame True {
                    n223 = call "获取最近两组水样测试数据.vi"("table"="CODCr") -> ("error out"=w456:errorcluster, "存储变量"=w457:T12)  [unwired: 9 in]
                    n224 = call "集成干预测试数据存储.vi"("error in (no error)"=w456, "存储变量"=w457) -> ()  [unwired: 9 in, 1 out]
                  }
                }
                n225 = case shown="真" w398 {
                  frame False {
                  }
                  frame True {
                    n226 = global read "断电保存变量.vi" "Temp"() -> (w415:bool)
                    n227 = case shown="真" w415 {
                      tunnel: [_ w452] -> w421
                      frame False {
                      }
                      frame True {
                        n228 = call "获取最近两组水样测试数据.vi"("table"="水温") -> ("error out"=w455:errorcluster, "存储变量"=w454:T12)  [unwired: 9 in]
                        n229 = call "集成干预测试数据存储.vi"("error in (no error)"=w455, "存储变量"=w454) -> ("error out"=w452:errorcluster)  [unwired: 9 in]
                      }
                    }
                    n230 = global read "断电保存变量.vi" "pH"() -> (w414:bool)
                    n231 = case shown="真" w414 {
                      tunnel: [_ w448] -> w420
                      tunnel: w421 -> [_ w447]
                      frame False {
                      }
                      frame True {
                        n232 = call "获取最近两组水样测试数据.vi"("error in (no error)"=w447, "table"="pH") -> ("error out"=w451:errorcluster, "存储变量"=w450:T12)  [unwired: 8 in]
                        n233 = call "集成干预测试数据存储.vi"("error in (no error)"=w451, "存储变量"=w450) -> ("error out"=w448:errorcluster)  [unwired: 9 in]
                      }
                    }
                    n234 = global read "断电保存变量.vi" "DO"() -> (w413:bool)
                    n235 = case shown="真" w413 {
                      tunnel: [_ w443] -> w419
                      tunnel: w420 -> [_ w442]
                      frame False {
                      }
                      frame True {
                        n236 = call "获取最近两组水样测试数据.vi"("error in (no error)"=w442, "table"="DO") -> ("error out"=w446:errorcluster, "存储变量"=w445:T12)  [unwired: 8 in]
                        n237 = call "集成干预测试数据存储.vi"("error in (no error)"=w446, "存储变量"=w445) -> ("error out"=w443:errorcluster)  [unwired: 9 in]
                      }
                    }
                    n238 = global read "断电保存变量.vi" "Cond"() -> (w412:bool)
                    n239 = case shown="真" w412 {
                      tunnel: [_ w438] -> w418
                      tunnel: w419 -> [_ w437]
                      frame False {
                      }
                      frame True {
                        n240 = call "获取最近两组水样测试数据.vi"("error in (no error)"=w437, "table"="比电导率") -> ("error out"=w441:errorcluster, "存储变量"=w440:T12)  [unwired: 8 in]
                        n241 = call "集成干预测试数据存储.vi"("error in (no error)"=w441, "存储变量"=w440) -> ("error out"=w438:errorcluster)  [unwired: 9 in]
                      }
                    }
                    n242 = global read "断电保存变量.vi" "Turb"() -> (w411:bool)
                    n243 = case shown="真" w411 {
                      tunnel: [_ w433] -> w417
                      tunnel: w418 -> [_ w432]
                      frame False {
                      }
                      frame True {
                        n244 = call "获取最近两组水样测试数据.vi"("error in (no error)"=w432, "table"="浊度") -> ("error out"=w436:errorcluster, "存储变量"=w435:T12)  [unwired: 8 in]
                        n245 = call "集成干预测试数据存储.vi"("error in (no error)"=w436, "存储变量"=w435) -> ("error out"=w433:errorcluster)  [unwired: 9 in]
                      }
                    }
                    n246 = global read "断电保存变量.vi" "叶绿素a启用"() -> (w410:bool)
                    n247 = case shown="真" w410 {
                      tunnel: [_ w428] -> w416
                      tunnel: w417 -> [_ w427]
                      frame False {
                      }
                      frame True {
                        n248 = call "获取最近两组水样测试数据.vi"("error in (no error)"=w427, "table"="叶绿素") -> ("error out"=w431:errorcluster, "存储变量"=w430:T12)  [unwired: 8 in]
                        n249 = call "集成干预测试数据存储.vi"("error in (no error)"=w431, "存储变量"=w430) -> ("error out"=w428:errorcluster)  [unwired: 9 in]
                      }
                    }
                    n250 = case shown="真" FALSE {
                      tunnel: [_ w423] -> _
                      tunnel: w416 -> [_ w422]
                      frame False {
                      }
                      frame True {
                        n251 = call "获取最近两组水样测试数据.vi"("error in (no error)"=w422, "table"="藻密度") -> ("error out"=w426:errorcluster, "存储变量"=w425:T12)  [unwired: 8 in]
                        n252 = call "集成干预测试数据存储.vi"("error in (no error)"=w426, "存储变量"=w425) -> ("error out"=w423:errorcluster)  [unwired: 9 in]
                      }
                    }
                  }
                }
              }
            }
          }
        }
        n253 = global read "采配水全局变量.vi" "状态"() -> (w310:T8)
        n254 = Unbundle By Name(w310) -> ("R0"=w309:i16)
        n255 = Equal To 0?(x=w309) -> (x = 0?=w308:bool)
        n256 = Select(t=enum16{"初始化", "采配水启动", "仪器操作", "反冲洗", "结束"}."结束" ("枚举"), s=w308, f=enum16{"初始化", "采配水启动", "仪器操作", "反冲洗", "结束"}."反冲洗" ("枚举")) -> (s? t:f=w305:enum16{"初始化", "采配水启动", "仪器操作", "反冲洗", "结束"})
      }
      frame "结束" {
        n257 = Release Queue(queue=w473) -> ()  [unwired: 2 in, 3 out]
        n258 = Unbundle By Name(w470) -> ("测试模式"=w471:enum16{"正常测试", "集成干预"})
        n259 = Cancel Notification(0:w474) -> (8:w475:refnum<notifier>)  [unwired: 1 in, 2 out]
        n260 = Release Notifier(notifier=w475) -> ()  [unwired: 2 in, 3 out]
        n261 = case shown="\"集成干预\"" w471 {
          tunnel: w469 -> [_ w478]
          frame "正常测试", Default {
          }
          frame "集成干预" {
            n262 = global write "系统设置全局变量.vi" "运行模式"(w478) -> ()
          }
        }
      }
    }
    n263 = Format Into String(format string="%s,当前运行时间%d秒" ("格式字符串"), w15, w11) -> (resulting string=w16:string)  [unwired: 2 in, 1 out]
    n264 = global write "采配水全局变量.vi" "运行状态显示"(w16) -> ()
  }
